vi "Start Test.vi"(0 "Candidate ID":string, 11 "error in (no error)":errorcluster) -> (4 "Started":bool, 15 "error out":errorcluster)   [LabVIEW 2014, in "Coding Platform.lvlib"]
uses:
  Coding Platform.lvlib
  Typedefs/User Event Operations.ctl
  Datatypes/Start Test.ctl
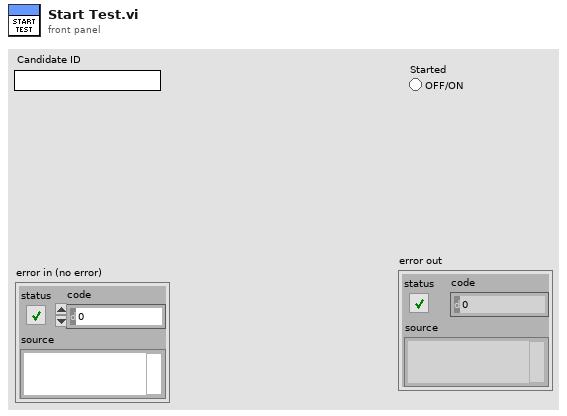
[diagram p1: front panel]
types:
  T1 = typedef "Coding Platform.lvlib/Start Test.ctl" = cluster{"Candidate_ID":string, "notifier":refnum<notifier>}
  T2 = typedef "Coding Platform.lvlib/User Event Operations.ctl" = enum16{"Create", "Genereate", "Destroy", "Get Reference"}
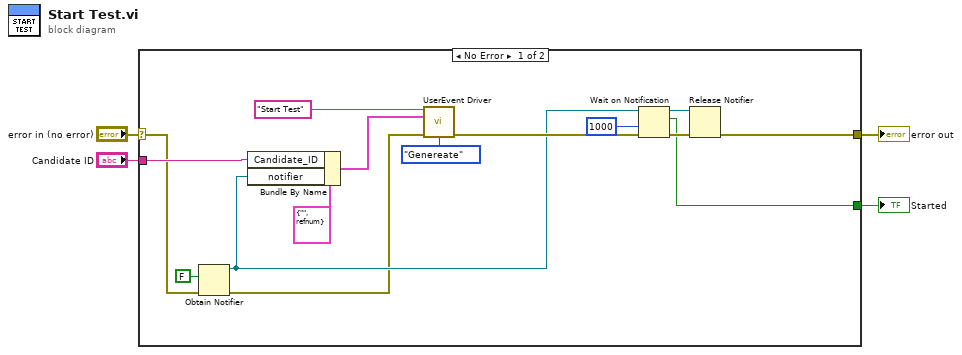
[diagram p0: block diagram]
diagram:
  n1 = case shown="No Error" "error in (no error)" {
    selector: "error in (no error)" -> [w5 w20]
    tunnel: [w9 w20] -> w4
    tunnel: "Candidate ID" -> [w14 _]
    tunnel: [w7 _] -> w1
    frame No Error {
      n2 = Obtain Notifier(notification data type=FALSE, error in (no error)=w5) -> (notifier out=w12:refnum<notifier>, error out=w6:errorcluster)  [unwired: 2 in, 1 out]
      n3 = Bundle By Name(cluster=T1 {"Candidate_ID"="", "notifier"=refnum} ("Login"), "Candidate_ID"=w14, "notifier"=w12) -> (w15:T1)
      n4 = call "UserEvent Driver.vi"("Message"="Start Test", "Data"=w15, "error in (no error)"=w6, "Operations(Get Reference)"=User_Event_Operations."Genereate") -> ("error out"=w19:errorcluster)  [unwired: 10 in, 1 out]
      n5 = Wait on Notification(notifier=w12, timeout in ms (-1)=1000, error in (no error)=w19) -> (notifier out=w8:refnum<notifier>, notification=w7:bool, error out=w13:errorcluster)  [unwired: 1 in, 1 out]
      n6 = Release Notifier(notifier=w8, error in (no error)=w13) -> (error out=w9:errorcluster)  [unwired: 1 in, 2 out]
    }
    frame Error {
    }
  }
  "error out" <- w4
  "Started" <- w1
